vi "PhotonCamera_SetPipelineIndex.vi"(9 "PipelineIndex":i32, 10 "BaseNTName":string="/photonvision", 11 "CameraName":string) -> (0 "error out":errorcluster)   [LabVIEW 2019, in "PhotonVisionLib.lvlib"]
doc: "Allows the user to select the active pipeline index.\n \nInputs:\n - cameraName -- The nickname of the camera (found in the PhotonVision UI).\n - index The active pipeline index.\n\nOutputs:\n - >none<"
uses:
  PhotonVisionLib.lvlib
  <vilib>/Rock Robotics/WPI/ThirdParty/JAS_Junk/TrajLib/VI/Util_GetTime_U32.vi
  <vilib>/Rock Robotics/WPI/ThirdParty/JAS_Junk/TrajLib/VI/Util_GetTime_U64.vi
  <vilib>/Rock Robotics/Network Tables/NT Read Integer.vi
  <vilib>/Rock Robotics/Network Tables/NT Write Integer.vi
  <vilib>/Rock Robotics/WPI/ThirdParty/JAS_Junk/TrajLib/Trajectory_Library.lvlib
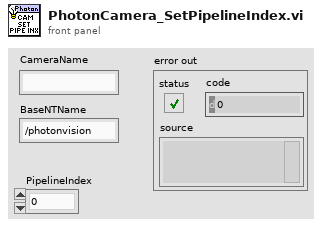
[diagram p1: front panel]
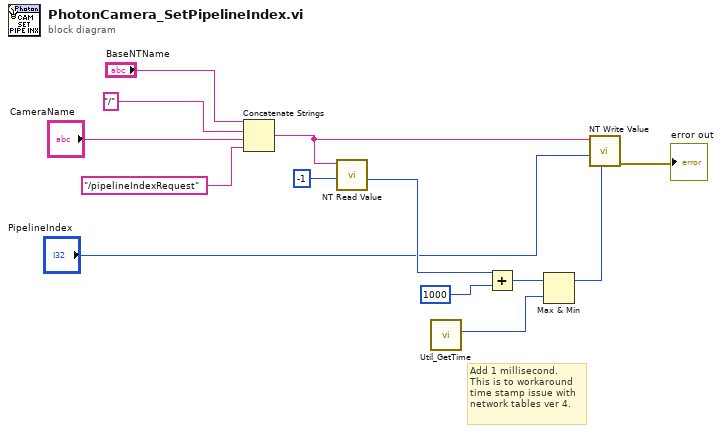
[diagram p0: block diagram]
diagram:
  # "Add 1 millisecond.\nThis is to workaround\ntime stamp issue with\nnetwork tables ver 4."
  n1 = Concatenate Strings("BaseNTName", "/", "CameraName", "/pipelineIndexRequest") -> (w4:string)
  n2 = call-poly <vilib>:"NT Read Value.vi"("default value"=i64 -1 ("Default Value"), "name"=w4) -> ("timestamp"=w6:u64)  [unwired: 7 in, 2 out]
  n3 = call <vilib>:"Util_GetTime.vi"() -> ("FPGA_Time_MicroSeconds"=w8:u64)  [unwired: 9 in, 2 out]
  n4 = Add(x=w6, y=u64 1000) -> (x+y=w9:u64)
  n5 = Max & Min(x=w9, y=w8) -> (max(x,y)=w5:u64)  [unwired: 1 out]
  n6 = call-poly <vilib>:"NT Write Value.vi"("timestamp"=w5, "value"="PipelineIndex", "name"=w4) -> ("error out"=→"error out":errorcluster)  [unwired: 8 in]
